vi "Időtömb.vi"(10 "Index":i32, 11 "Bemeneti tömb":string[](array[string])) -> (2 "Perc":dbl, 3 "Óra":dbl)   [LabVIEW 2014]
doc: "A bemeneti tömböt elemeire bontja (az indexeket az index értékbe kell bevezeni) tömbre bontja fel ez a SubVI .\nAz így kapott szöveget egy tömbre bontja fel, és a két oszlop értékeit a kettõspont választja el egymástól.\n\nCiklusban ajánlatos alkalmazni, a bemeneti tömb óra:perc felépítésû értékeinek szétválogatására külön órára, és percre."
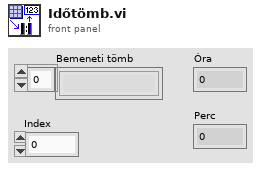
[diagram p1: front panel]
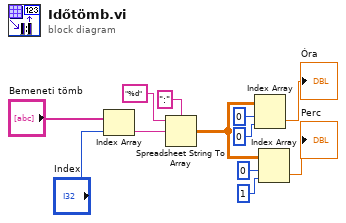
[diagram p0: block diagram]
diagram:
  n1 = Index Array(array="Bemeneti tömb", index="Index") -> (element=w10:string)
  n2 = Spreadsheet String To Array(delimiter (Tab)=":", format string="%d", spreadsheet string=w10) -> (array=w7:dbl[][])  [unwired: 1 in]
  n3 = Index Array(array=w7, index (row)=0, index (col)=0 ("disabled index (col)")) -> (element=→"Óra":dbl)
  n4 = Index Array(array=w7, index (row)=0, index (col)=1 ("disabled index (col)")) -> (element=→"Perc":dbl)
